vi "data_processing_loop.vi"(11 "Message Queues":T1) -> ()   [LabVIEW 2017, in "data_processing.lvlib"]
uses:
  data_processing.lvlib
  support/Message Queue/All Message Queues.ctl
  support/Message Queue/Message Cluster.ctl
  support/Message Queue/Message Queue.lvlib
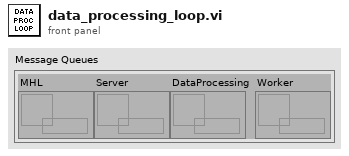
[diagram p1: front panel]
types:
  T1 = typedef "Message Queue.lvlib/All Message Queues.ctl" = cluster{"MHL":refnum<queue>, "Server":refnum<queue>, "DataProcessing":refnum<queue>, "Worker":refnum<queue>}
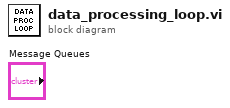
[diagram p0: block diagram]
diagram:
